vi "Items Mouse Click.vi"(6 "PlatMods":T1, 7 "Mods":cluster{"Double Click":bool, "Menu Key":bool}, 8 "error in (no error)":errorcluster, 9 "Button":u16, 10 "Coords":T2, 11 "Sequence Element in":refnum<class "Sequence Element.lvclass">) -> (0 "error out":errorcluster, 1 "Valid":bool, 2 "Name":string, 3 "Sequence Element out":refnum<class "Sequence Element.lvclass">, 4 "Double click":bool, 5 "In symbol":bool)   [LabVIEW 2016, in "Sequence Element.lvclass"]
uses:
  Sequence Element.lvclass
  <vilib>/Utility/miscctls.llb/LVPoint32TypeDef.ctl
  Sequence Element.lvclass/Sequence Element.ctl
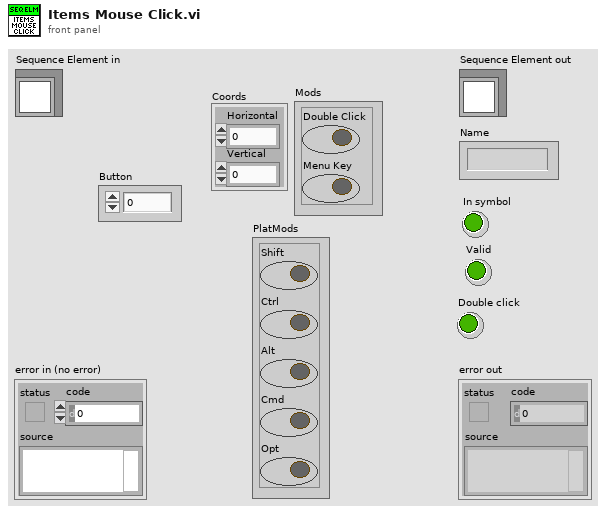
[diagram p1: front panel]
types:
  T1 = cluster{"Shift":bool, "Ctrl":bool, "Alt":bool, "Cmd":bool, "Opt":bool}
  T2 = typedef "LVPoint32TypeDef.ctl" = cluster{"Horizontal":i32, "Vertical":i32}
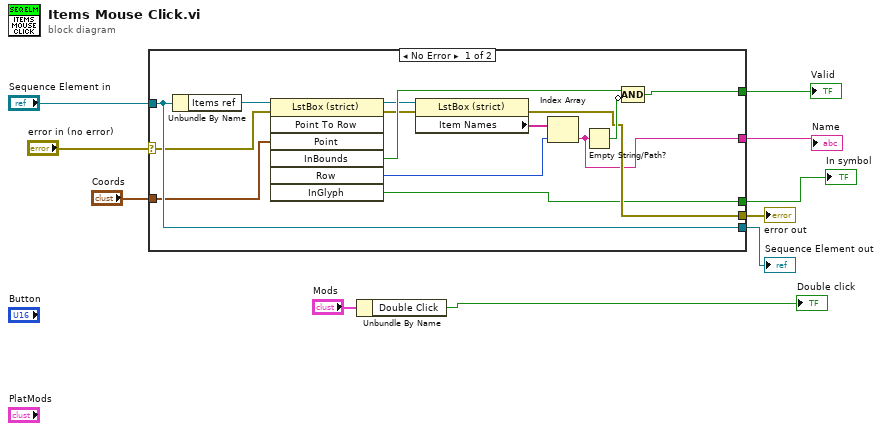
[diagram p0: block diagram]
diagram:
  n1 = case shown="No Error" "error in (no error)" {
    selector: "error in (no error)" -> [w16 w26]
    tunnel: [w15 w26] -> w9
    tunnel: [w24 w25] -> w7
    tunnel: "Sequence Element in" -> [w24 w25]
    tunnel: "Coords" -> [w23 _]
    tunnel: [w14 _] -> w5
    tunnel: [w13 _] -> w4
    tunnel: [w12 _] -> w3
    frame No Error {
      n2 = Unbundle By Name(w24) -> ("Items ref"=w11:refnum<vi>)
      n3 = invoke class="LstBox (strict)" method="Point To Row"(reference=w11, error in=w16, "Point"=w23) -> (reference out=w21:refnum<vi>, error out=w20:errorcluster, "InBounds"=w22:bool, "Row"=w18:i32, "InGlyph"=w13:bool)  [unwired: 4 in, 2 out]
      n4 = property class="LstBox (strict)"(reference=w21, error in=w20) -> (error out=w15:errorcluster, "Item Names"=w19:string[])  [unwired: 1 out]
      n5 = Index Array(array=w19, index=w18) -> (element=w14:string)
      n6 = Empty String/Path?(string/path=w14) -> (empty?=w17:bool)
      n7 = Compound Arithmetic op=AND(w22, invert w17) -> (w12:bool)
    }
    frame Error {
    }
  }
  "error out" <- w9
  "Sequence Element out" <- w7
  "Name" <- w5
  "In symbol" <- w4
  "Valid" <- w3
  n8 = Unbundle By Name("Mods") -> ("Double Click"=→"Double click":bool)
